vi "Test Snake Grows only Once After Eating.vi"(8 "error in (no error)":errorcluster, 11 "Test Case In":refnum<class "Snake Test.lvclass">) -> (0 "error out":errorcluster, 3 "Test Case Out":refnum<class "Snake Test.lvclass">)   [LabVIEW 2020, in "Snake Test.lvclass"]
uses:
  Snake Test.lvclass
  C:/Program Files (x86)/National Instruments/LabVIEW 2020/vi.lib/Astemes/LUnit/Test Case.lvclass
  source/Snake/Direction.ctl
  source/Particle/Position.ctl
  <vilib>/Astemes/LUnit/Test Case.lvclass/Test Case.ctl
  <vilib>/Astemes/LUnit/Set Assertion Type.vi
  <vilib>/Astemes/LUnit/Palette/Pass.vi
  <vilib>/Astemes/LUnit/Palette/Fail.vi
  <vilib>/Astemes/LUnit/Add test result.vi
  <vilib>/Astemes/LUnit/LUnit Record Assertion Result.vi
  <vilib>/Astemes/LUnit/LUnit Aggregate Assertion Results.vi
  <vilib>/Astemes/LUnit/Method Result/LUnit Merge Status.vi
  <vilib>/Astemes/LUnit/LUnit Concatenate result strings.vi
  source/Snake/Snake.lvclass
  source/Particle.lvclass
  <vilib>/Astemes/LUnit/Test Case.lvclass
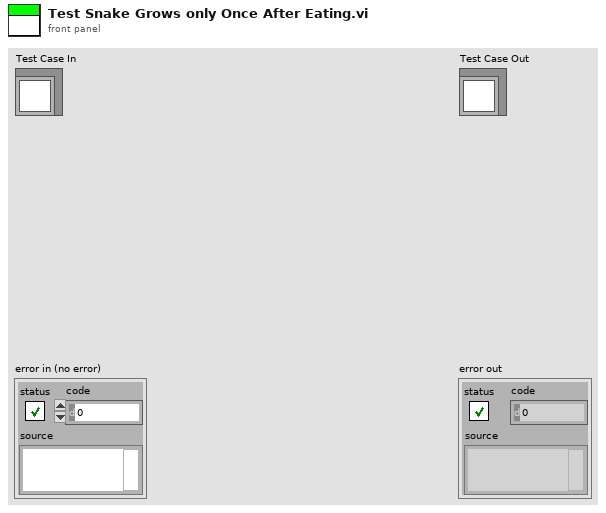
[diagram p1: front panel]
types:
  T1 = typedef "Particle.lvclass/Position.ctl" = cluster{"X":i32, "Y":i32}
  T2 = typedef "Snake.lvclass/Direction.ctl" = enum16{"X", "-X", "Y", "-Y"}
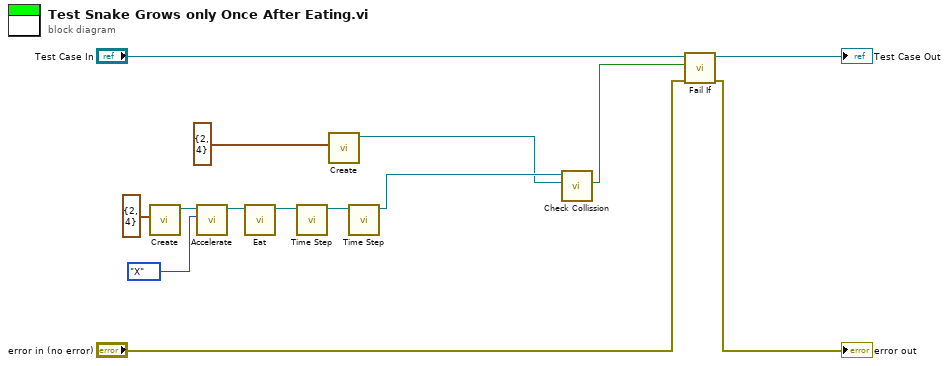
[diagram p0: block diagram]
diagram:
  n1 = call "Create.vi"("Position"=T1 {"X"=2, "Y"=4}) -> ("Snake out"=w10:refnum<class "Snake.lvclass">)  [unwired: 10 in]
  n2 = call "Accelerate.vi"("Direction"=Direction."X", "Snake in"=w10) -> ("Snake out"=w7:refnum<class "Snake.lvclass">)  [unwired: 9 in]
  n3 = call "Eat.vi"("Snake in"=w7) -> ("Snake out"=w8:refnum<class "Snake.lvclass">)  [unwired: 10 in]
  n4 = call "Time Step.vi"("Snake in"=w8) -> ("Snake out"=w1:refnum<class "Snake.lvclass">)  [unwired: 10 in]
  n5 = call "Create.vi"("Position"=T1 {"X"=2, "Y"=4}) -> ("Particle out"=w3:refnum<class "Particle.lvclass">)  [unwired: 10 in]
  n6 = call "Time Step.vi"("Snake in"=w1) -> ("Snake out"=w5:refnum<class "Snake.lvclass">)  [unwired: 10 in]
  n7 = call "Check Collission.vi"("Particle"=w3, "Snake in"=w5) -> ("Collided?"=w2:bool)  [unwired: 8 in, 1 out]
  n8 = call <vilib>:"Fail If.vi"("error in (no error)"="error in (no error)", "Fail?"=w2, "LUnit Test Case In"="Test Case In") -> ("error out"=→"error out":errorcluster, "LUnit Test Case Out"=→"Test Case Out":refnum<class "Snake Test.lvclass">)  [unwired: 7 in]
